vi "To Serial Form.vi"(6 "Serial Version":T1, 10 "Serializer in":refnum<class "Serializer.lvclass">, 11 "CRDS Data in":refnum<class "CRDS Data.lvclass">) -> (0 "error out":errorcluster, 2 "Serializer out":refnum<class "Serializer.lvclass">, 3 "CRDS Data out":refnum<class "CRDS Data.lvclass">)   [LabVIEW 2014, in "CRDS Data.lvclass"]
uses:
  CRDS Data.lvclass
  <vilib>/NI/AQ Character Lineator/Serializer/Serializer.lvclass
  <vilib>/NI/AQ Character Lineator/Serialization Common/Serial Version.ctl
  Cell/CRDS Cell Data.lvclass
  CRDS Data.lvclass/CRDS Data.ctl
  <vilib>/NI/AQ Character Lineator/Serializable/Insert Boolean.vi
  <vilib>/NI/AQ Character Lineator/Serializable/Insert Single.vi
  <vilib>/NI/AQ Character Lineator/Serializable/Insert Serializable Array.vi
  <vilib>/NI/AQ Character Lineator/Serializer/Insert Boolean.vi
  <vilib>/NI/AQ Character Lineator/Serializer/Insert Single.vi
  <vilib>/NI/AQ Character Lineator/Serializer/Read Include Default Values.vi
  <vilib>/NI/AQ Character Lineator/Serializer/Insert Serializable Array.vi
  Data/Data.lvclass
  <vilib>/NI/AQ Character Lineator/Serializable/Serializable.lvclass
  <vilib>/NI/AQ Character Lineator/Serialization Common/Serialization Common.lvlib
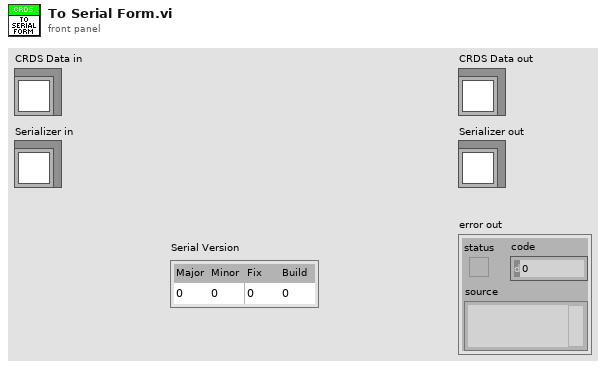
[diagram p1: front panel]
types:
  T1 = typedef "Serialization Common.lvlib/Serial Version.ctl" = cluster{"Major":u16, "Minor":u16, "Fix":u16, "Build":u16}
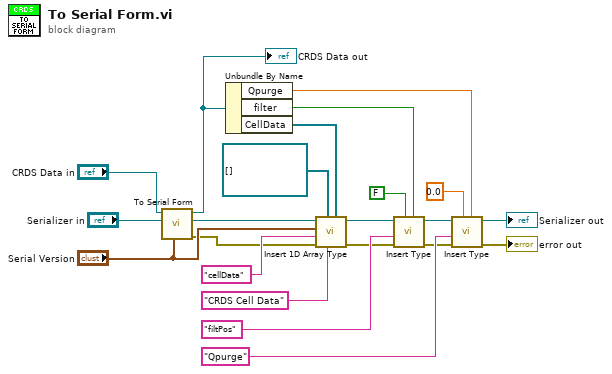
[diagram p0: block diagram]
diagram:
  n1 = call-parent "To Serial Form.vi"("Serial Version"="Serial Version", "Serializer in"="Serializer in", "Data in"="CRDS Data in") -> ("error out"=w1:errorcluster, "Serializer out"=w7:refnum<class "Serializer.lvclass">, "Data out"=w20:refnum<class "CRDS Data.lvclass">)  [unwired: 6 in]
  "CRDS Data out" <- w20
  n2 = Unbundle By Name(w20) -> ("Qpurge"=w13:sgl, "filter"=w19:bool, "CellData"=w8:refnum<class "CRDS Cell Data.lvclass">[])
  n3 = call-poly <vilib>:"Insert 1D Array Type.vi"("Serializables"=w8, "Default Class Qualified Name"="CRDS Cell Data", "Default Value"=refnum<class "CRDS Cell Data.lvclass">[] [] ("CellData"), "error in (no error)"=w1, "Name"="cellData", "Serial Version"="Serial Version", "Serializer in"=w7) -> ("error out"=w2:errorcluster, "Serializer out"=w3:refnum<class "Serializer.lvclass">)  [unwired: 3 in]
  n4 = call-poly <vilib>:"Insert Type.vi"("Boolean"=w19, "Default Value"=FALSE, "error in (no error)"=w2, "Name"="filtPos", "Serializer in"=w3) -> ("error out"=w11:errorcluster, "Serializer out"=w16:refnum<class "Serializer.lvclass">)  [unwired: 5 in]
  n5 = call-poly <vilib>:"Insert Type.vi"("Double"=w13, "Default Value"=sgl 0.0, "error in (no error)"=w11, "Name"="Qpurge", "Serializer in"=w16) -> ("error out"=→"error out":errorcluster, "Serializer out"=→"Serializer out":refnum<class "Serializer.lvclass">)  [unwired: 5 in]
